vi "data insert.vi"(8 "error in (no error)":errorcluster, 10 "data in":T1={"时间"=timestamp(0 s since 1904-01-01), "测量模式"="", "数据类型"="N", "水样实测值"=0.0, "单位"="", "水样数据标识"="N", "信号值"=0.0, "标样参考值"=0.0, "因子编码"="", "探头温度"=0.0}, 11 "table in":string(combo)) -> (0 "error out":errorcluster)   [LabVIEW 2016, in "斯坦道多参数.lvlib"]
uses:
  <vilib>/addons/database/Auxilliary.llb/DB Tools Column Info.ctl
  <vilib>/addons/database/Auxilliary.llb/DB Tools DataTypes.ctl
  <vilib>/addons/database/NI_Database_API.lvlib
  WxMessage/wxpusher.lvlib
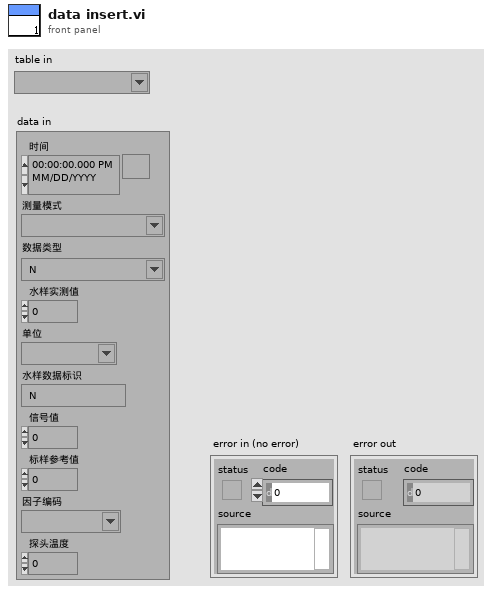
[diagram p1: front panel]
types:
  T1 = cluster{"时间":timestamp, "测量模式":string, "数据类型":string, "水样实测值":sgl, "单位":string, "水样数据标识":string, "信号值":sgl, "标样参考值":sgl, "因子编码":string, "探头温度":sgl}
  T2 = typedef "NI_Database_API.lvlib/DB Tools Column Info.ctl" = cluster{"column name":string, "data type":T3, "size":i32, "allow null?":bool}
  T3 = typedef "NI_Database_API.lvlib/DB Tools DataTypes.ctl" = enum16{"String", "Long (I32)", "Single (SGL)", "Double (DBL)", "Date/Time", "Binary"}
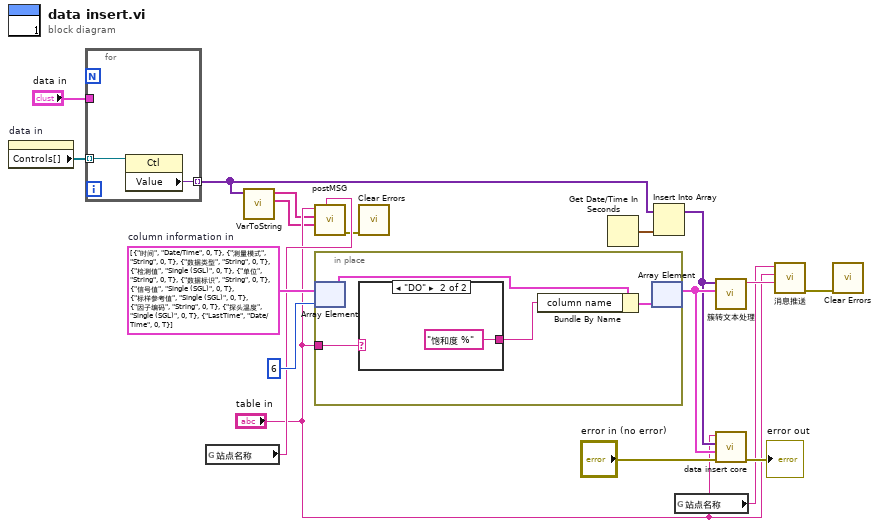
[diagram p0: block diagram]
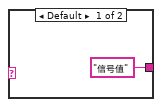
[diagram p2: hidden frame]
diagram:
  w12 = T2[] [{"column name"="时间", "data type"=enum."Date/Time", "size"=0, "allow null?"=TRUE}, {"column name"="测量模式", "data type"=enum."String", "size"=0, "allow null?"=TRUE}, {"column name"="数据类型", "data type"=enum."String", "size"=0, "allow null?"=TRUE}, {"column name"="检测值", "data type"=enum."Single (SGL)", "size"=0, "allow null?"=TRUE}, {"column name"="单位", "data type"=enum."String", "size"=0, "allow null?"=TRUE}, {"column name"="数据标识", "data type"=enum."String", "size"=0, "allow null?"=TRUE}, {"column name"="信号值", "data type"=enum."Single (SGL)", "size"=0, "allow null?"=TRUE}, {"column name"="标样参考值", "data type"=enum."Single (SGL)", "size"=0, "allow null?"=TRUE}, {"column name"="因子编码", "data type"=enum."String", "size"=0, "allow null?"=TRUE}, {"column name"="探头温度", "data type"=enum."Single (SGL)", "size"=0, "allow null?"=TRUE}, {"column name"="LastTime", "data type"=enum."Date/Time", "size"=0, "allow null?"=TRUE}]  # column information in
  n1 = property on="data in" class="Clust (严格)"() -> ("Controls[]"=w18:refnum<vi>[])  [unwired: 2 in, 2 out]
  n2 = for {
    tunnel: w18 -> [w20] mode=indexing
    tunnel: [w19] -> w5 mode=indexing
    tunnel: "data in" -> [_]
    n3 = property class="Ctl"(reference=w20) -> ("Value"=w19:variant)  [unwired: 1 in, 2 out]
  }
  n4 = global read "系统设置全局变量.vi" "站点名称"() -> (w7:string)
  n5 = call "VarToString.vi"("数组"=w5) -> ("data"=w3:string[], "columns"=w4:string[])  [unwired: 9 in]
  n6 = call "postMSG.vi"("station"=w7, "data"=w3, "columns"=w4, "table"="table in") -> ("error out"=w1:errorcluster)  [unwired: 7 in]
  n7 = in-place {
    in-place-border: "table in" -> [w24]
    n8 = in-place-array #1(w12, 6) -> (w21:T2)
    n9 = case shown="\"DO\"" w24 {
      tunnel: ["信号值" ("column name") "饱和度 %" ("column name")] -> w23
      frame Default {
      }
      frame "DO" {
      }
    }
    n10 = Bundle By Name(cluster=w21, "column name"=w23) -> (w22:T2)
    n11 = in-place-array #1(w22) -> (w9:T2[])  [unwired: 1 out]
  }
  n12 = call <vilib>:"Clear Errors.vi"("error in (no error)"=w1) -> ()  [unwired: 5 in, 2 out]
  n13 = Get Date/Time In Seconds() -> (seconds since 1Jan1904=w16:timestamp)
  n14 = Insert Into Array(array=w5, new element=w16) -> (w8:variant[])  [unwired: 1 in]
  n15 = global read "系统设置全局变量.vi" "站点名称"() -> (w10:string)
  n16 = call "簇转文本处理.vi"("column information"=w9, "data"=w8) -> ("output"=w11:string)  [unwired: 9 in]
  n17 = call "data insert core.vi"("error in (no error)"="error in (no error)", "column information"=w9, "data"=w8, "table"="table in") -> ("error out"=→"error out":errorcluster)  [unwired: 7 in]
  n18 = call "消息推送.vi"("分析"=w11, "内容"="table in", "站点"=w10) -> ("error out"=w2:errorcluster)  [unwired: 8 in]
  n19 = call <vilib>:"Clear Errors.vi"("error in (no error)"=w2) -> ()  [unwired: 5 in, 2 out]
